vi "Init Image.vi"(8 "error in (no error)":errorcluster, 11 "LF2R IDE in":refnum<class "Main Panel.lvclass">) -> (0 "error out":errorcluster, 3 "LF2R IDE out":refnum<class "Main Panel.lvclass">)   [LabVIEW 2018, in "Main Panel.lvlib" / "Main Panel.lvclass"]
uses:
  Main Panel.lvclass
  Main Panel.lvclass/Main Panel.ctl
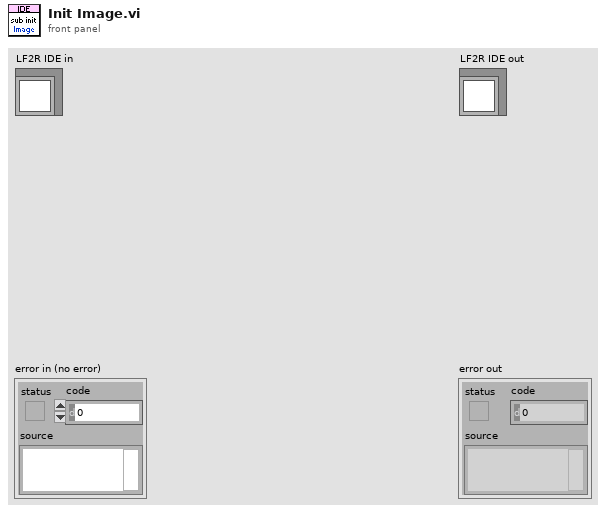
[diagram p1: front panel]
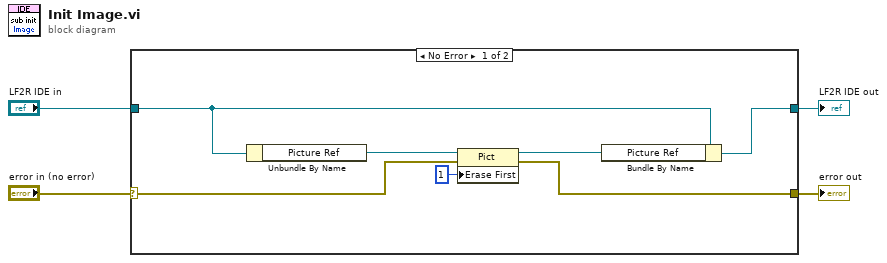
[diagram p0: block diagram]
diagram:
  n1 = case shown="No Error" "error in (no error)" {
    selector: "error in (no error)" -> [w10 w13]
    tunnel: [w8 w13] -> w3
    tunnel: [w5 w12] -> w1
    tunnel: "LF2R IDE in" -> [w7 w12]
    frame No Error {
      n2 = Unbundle By Name(w7) -> ("Picture Ref"=w11:refnum<vi>)
      n3 = property class="Pict"(reference=w11, error in=w10, "Erase First"=u8 1) -> (reference out=w6:refnum<vi>, error out=w8:errorcluster)
      n4 = Bundle By Name(cluster=w7, "Picture Ref"=w6) -> (w5:refnum<class "Main Panel.lvclass">)
    }
    frame Error {
    }
  }
  "error out" <- w3
  "LF2R IDE out" <- w1
